vi "process_watchdog.vi"() -> ()   [LabVIEW 2010]
uses:
  typedefs/data_cluster.ctl
  globals/exit.vi
panel:
  out "#":i32
  out "#":i32
  out "#":i32
  out "error out":errorcluster
  out "Data_to_analysis_queue":bool
  out "Data_to_display_queue":bool
  out "Data_to_storage_queue":bool
  in  "error in (no error)":errorcluster
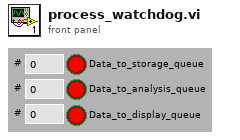
[diagram p1: front panel]
types:
  T1 = typedef "data_cluster.ctl" = cluster{"t0":dbl, "dt":dbl, "Channels":dbl[][]}
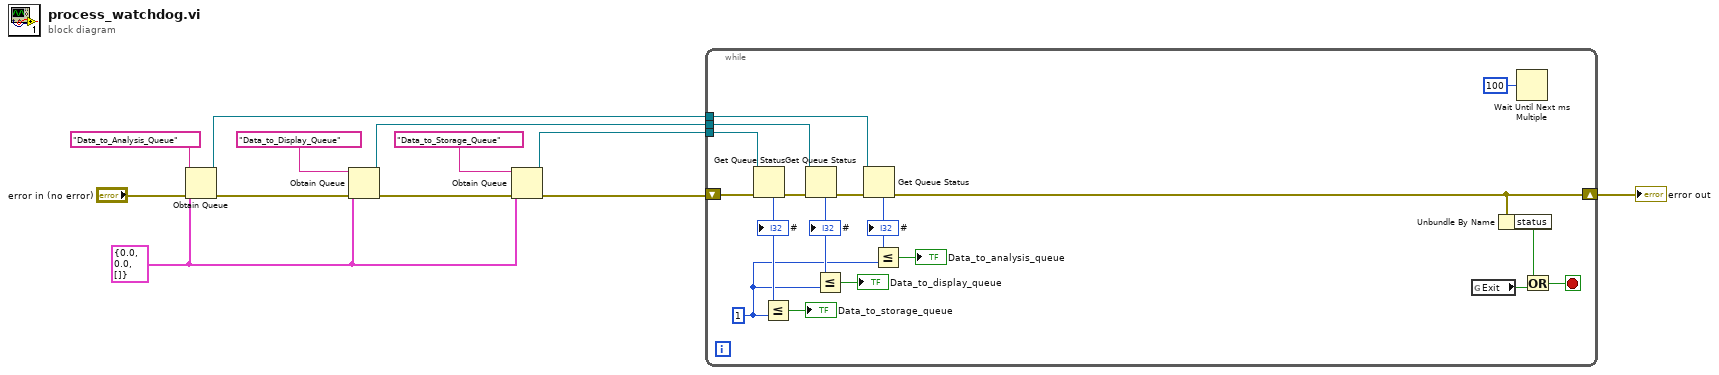
[diagram p0: block diagram]
diagram:
  w1 = T1 {"t0"=0.0, "dt"=0.0, "Channels"=[]} ("Data cluster")
  n1 = Obtain Queue(name (unnamed)="Data_to_Analysis_Queue", element data type=w1, error in (no error)="error in (no error)") -> (queue out=w6:refnum<queue>, error out=w9:errorcluster)  [unwired: 2 in, 1 out]
  n2 = Obtain Queue(name (unnamed)="Data_to_Display_Queue", element data type=w1, error in (no error)=w9) -> (queue out=w5:refnum<queue>, error out=w11:errorcluster)  [unwired: 2 in, 1 out]
  n3 = Obtain Queue(name (unnamed)="Data_to_Storage_Queue", element data type=w1, error in (no error)=w11) -> (queue out=w4:refnum<queue>, error out=w7:errorcluster)  [unwired: 2 in, 1 out]
  n4 = while {
    tunnel: w6 -> [w21]
    tunnel: w5 -> [w25]
    tunnel: w4 -> [w29]
    shift-right: [w13] -> w3
    shift-left: w7 -> [w30]
    stop <- w15 stop-if-true
    w18 = 1 ("y")
    n5 = Get Queue Status(queue=w29, error in (no error)=w30) -> (error out=w26:errorcluster, # elements in queue=w28:i32)  [unwired: 1 in, 6 out]
    "#" <- w28
    n6 = Less Or Equal?(x=w28, y=w18) -> (x <= y?=→"Data_to_storage_queue":bool)
    n7 = Get Queue Status(queue=w25, error in (no error)=w26) -> (error out=w22:errorcluster, # elements in queue=w23:i32)  [unwired: 1 in, 6 out]
    "#" <- w23
    n8 = Less Or Equal?(x=w23, y=w18) -> (x <= y?=→"Data_to_display_queue":bool)
    n9 = Get Queue Status(queue=w21, error in (no error)=w22) -> (error out=w13:errorcluster, # elements in queue=w19:i32)  [unwired: 1 in, 6 out]
    "#" <- w19
    n10 = Less Or Equal?(x=w19, y=w18) -> (x <= y?=→"Data_to_analysis_queue":bool)
    n11 = global read "exit.vi" "Exit"() -> (w14:bool)
    n12 = Unbundle By Name(w13) -> ("status"=w16:bool)
    n13 = Wait Until Next ms Multiple(millisecond multiple=u32 100) -> ()  [unwired: 1 out]
    n14 = Or(x=w16, y=w14) -> (x .or. y?=w15:bool)
  }
  "error out" <- w3
